vi "Write Syringe.vi"(8 "error in (no error)":errorcluster, 10 "Syringe":bool, 11 "Carrier Tray in":refnum<class "Assembly Tray.lvclass">) -> (0 "error out":errorcluster, 3 "Carrier Tray out":refnum<class "Assembly Tray.lvclass">)   [LabVIEW 2021, in "Assembly Tray.lvclass"]
uses:
  Assembly Tray.lvclass
  Assembly Tray.lvclass/Assembly Tray.ctl
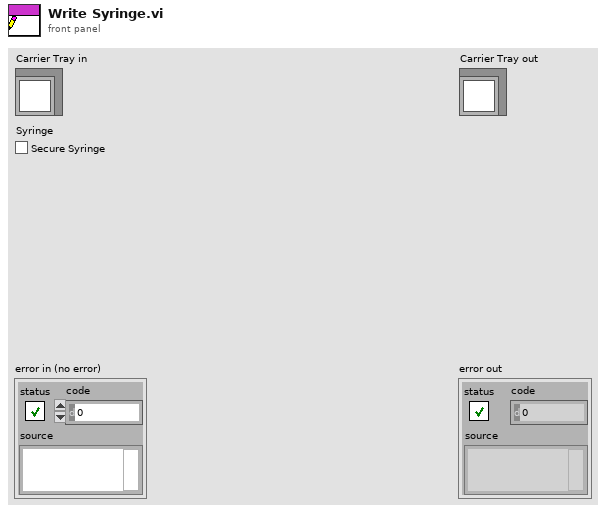
[diagram p1: front panel]
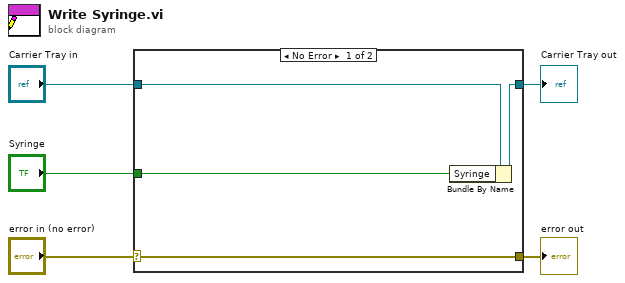
[diagram p0: block diagram]
diagram:
  n1 = case shown="No Error" "error in (no error)" {
    selector: "error in (no error)" -> [w9 w10]
    tunnel: [w9 w10] -> w4
    tunnel: [w7 w11] -> w2
    tunnel: "Carrier Tray in" -> [w8 w11]
    tunnel: "Syringe" -> [w6 _]
    frame No Error {
      n2 = Bundle By Name(cluster=w8, "Syringe"=w6) -> (w7:refnum<class "Assembly Tray.lvclass">)
    }
    frame Error {
    }
  }
  "error out" <- w4
  "Carrier Tray out" <- w2
